vi "Enqueue Read Multi-M.vi"(8 "Error In":errorcluster, 9 "Length (U16)":u16, 10 "Start Position (U32)":u32, 11 "Name":string) -> (0 "Error Out":errorcluster)   [LabVIEW 2019, in "FX5U SLMP Binary.lvlib"]
uses:
  FX5U SLMP Binary.lvlib
  Queue/Queue.lvlib
  Error Notifier/Error Notifier.lvlib
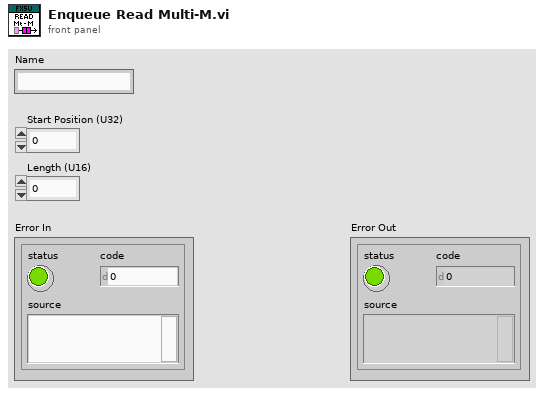
[diagram p1: front panel]
types:
  T1 = cluster{"Start Position (U32)":u32, "Length (U16)":u16}
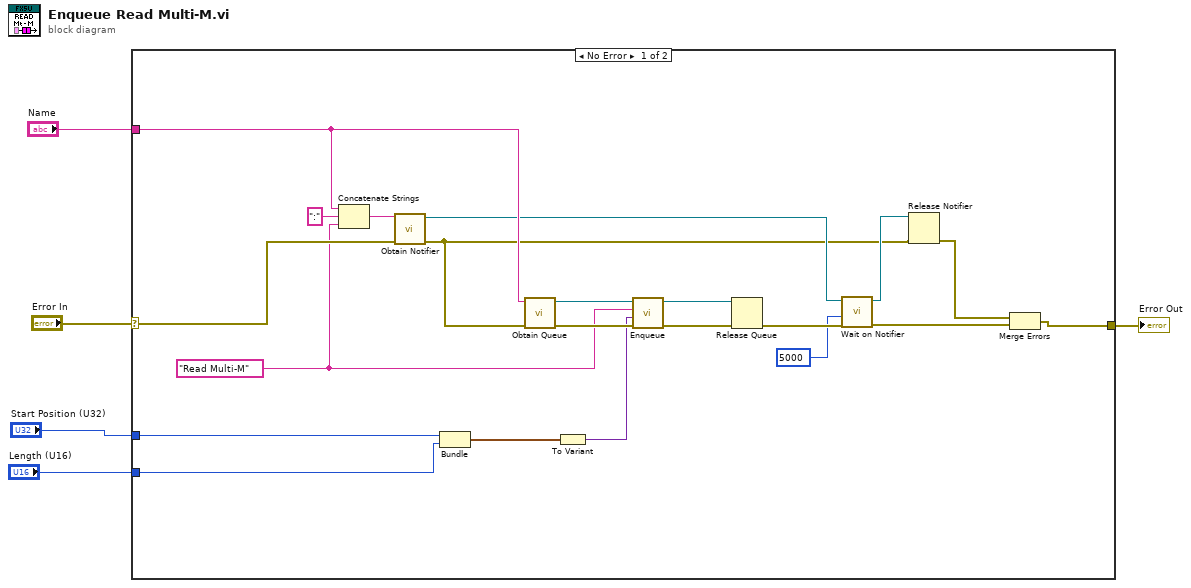
[diagram p0: block diagram]
diagram:
  n1 = case shown="No Error" "Error In" {
    selector: "Error In" -> [w26 w27]
    tunnel: [w11 w27] -> w4
    tunnel: "Name" -> [w24 _]
    tunnel: "Start Position (U32)" -> [w9 _]
    tunnel: "Length (U16)" -> [w8 _]
    frame No Error {
      w21 = "Read Multi-M" ("Message")
      n2 = Concatenate Strings(w24, ":" ("string"), w21) -> (w23:string)
      n3 = call "Obtain Notifier.vi"("Error In"=w26, "Name"=w23) -> ("Error Out"=w10:errorcluster, "notifier out"=w16:refnum<notifier>)  [unwired: 8 in]
      n4 = Bundle("Start Position (U32)"=w9, "Length (U16)"=w8) -> (w7:T1)  [unwired: 1 in]
      n5 = call "Obtain Queue.vi"("Error In"=w10, "Name"=w24) -> ("Error Out"=w25:errorcluster, "queue out"=w19:refnum<queue>)  [unwired: 8 in]
      n6 = To Variant(anything=w7) -> (Variant=w6:variant)
      n7 = call "Enqueue.vi"("Error In"=w25, "Data"=w6, "Message"=w21, "queue in"=w19) -> ("Error Out"=w20:errorcluster, "queue out"=w18:refnum<queue>)  [unwired: 6 in]
      n8 = Release Queue(queue=w18, error in (no error)=w20) -> (error out=w17:errorcluster)  [unwired: 1 in, 2 out]
      n9 = call "Wait on Notifier.vi"("Error In"=w17, "timeout in ms (-1)"=5000, "notifier in"=w16) -> ("Error Out"=w12:errorcluster, "notifier out"=w14:refnum<notifier>)  [unwired: 7 in]
      n10 = Release Notifier(notifier=w14, error in (no error)=w10) -> (error out=w13:errorcluster)  [unwired: 1 in, 2 out]
      n11 = Merge Errors(w13, w12) -> (w11:errorcluster)
    }
    frame Error {
    }
  }
  "Error Out" <- w4
